vi "Periodic Tasks.vi"(8 "error constant":errorcluster) -> ()   [LabVIEW 2014]
doc: "This VI runs in parallel to other tasks. It can contain as many user-defined periodic loops as you need. These can carry out PID or other sorts of timed response."
uses:
  <vilib>/Rock Robotics/WPI/Solenoid/WPI_SolenoidValue.ctl
  Dashboard Project/DashboardToRobotCluster.ctl
  Robot Global Data.vi
  <vilib>/Rock Robotics/WPI/Solenoid/WPI_SolenoidSetEnum.vi
  <vilib>/Rock Robotics/WPI/RobotDrive/WPI_RobotDriveGetSetRefNum.vi
  <vilib>/Rock Robotics/WPI/RobotDrive/WPI_RobotDriveMecanumDrive_Cartesian.vi
  navX-MXP Library/navX-MXP IMU.lvlib
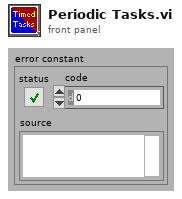
[diagram p1: front panel]
types:
  T1 = typedef "DashboardToRobotCluster.ctl" = cluster{"Test":dbl}
  T2 = typedef "WPI_SolenoidValue.ctl" = enum16{"Off", "On", "Forward", "Reverse"}
  T3 = cluster{"Front Right Motor":dbl, "Front Left Motor":dbl, "Rear Right Motor":dbl, "Rear Left Motor":dbl, "Current Heading":dbl, "Tote lift Up":bool, "Primary Feeder running":bool, "Secondary Feeder running":bool, "Totes In Robot":dbl, "Pressure In Tank":dbl, "Can Grabber State":T2}
  T4 = typedef "navX-MXP IMU.lvlib/navX SPI DevRef.ctl" = cluster{"SPIDevRef":T5, "Board Information":T8, "Status":T9, "Offsets":cluster{"Yaw":dbl, "Quat W":dbl, "Quat X":dbl, "Quat Y":dbl, "Quat Z":dbl}, "Update Rate (4Hz-60Hz)":u8, "refnum name":string, "error":errorcluster}
  T5 = typedef "WPI_SPIDevRef.ctl" = cluster{"DevStatus":errorcluster, "Handle":i32, "Controller":T6, "SPI Bus":T7}
  T6 = typedef "FPGA_TypedefDigitalModule.ctl" = enum16{"Controller 1"}
  T7 = typedef "spi_bus.ctl" = enum16{"SPI On-Board, CS0", "SPI On-Board, CS1", "SPI On-Board, CS2", "SPI On-Board, CS3", "SPI MXP", "Invalid"}
  T8 = typedef "navX-MXP IMU.lvlib/navX Board Information.ctl" = cluster{"WhoAmI (50 | 0x32)":u8, "Board Revision":u8, "Firmware Major Version":u8, "Firmware Minor Version":u8}
  T9 = typedef "navX-MXP IMU.lvlib/navX Status Data.ctl" = cluster{"Update Rate Hz":u8, "Accelerometer Full-Scale Range":u8, "Gyro Full-Scale Range":u16, "NAVX_OP_STATUS":T10, "NAVX_CAL_STATUS":T11, "NAVX_SELFTEST_STATUS":u8, "NAVX_SENSOR_STATUS":T12}
  T10 = typedef "navX-MXP IMU.lvlib/navX NAVX_OP_STATUS.ctl" = u8
  T11 = typedef "navX-MXP IMU.lvlib/navX NAVX_CAL_STATUS.ctl" = u8
  T12 = typedef "navX-MXP IMU.lvlib/navX NAVX_SENSOR_STATUS.ctl" = cluster{"MOVING":bool, "YAW_STABLE":bool, "MAG_DISTURBANCE":bool, "ALTITUDE_VALID":bool, "SEALEVEL_PRESS_SET":bool, "FUSED_HEADING_VALID":bool}
  T13 = typedef "WPI_RobotDriveDevRef.ctl" = cluster{"DevStatus":errorcluster, "Motors[]":T14[], "Square Inputs":bool, "Max Output":dbl}
  T14 = typedef "WPI_MotorControlDeviceRef.ctl" = cluster{"DeviceStatus":errorcluster, "Type":T15, "PWM":cluster{"Controller":T6, "PWM Channel":T16, "DeadBand":T17}, "CAN":cluster{"Device Number":u8, "Control Mode":T18, "Semaphore":T19, "Max Vout":dbl, "TalonSRX Control Mode":T20}, "Invert":bool, "TransformRef":T21, "InvTransformRef":T21}
  T15 = typedef "WPI_MotorControlType.ctl" = enum16{"PWM", "CAN", "CANTalonSRX"}
  T16 = typedef "FPGA_DIOPWMChannel.ctl" = enum8{"PWM 0", "PWM 1", "PWM 2", "PWM 3", "PWM 4", "PWM 5", "PWM 6", "PWM 7", "PWM 8", "PWM 9", "PWM MXP 0", "PWM MXP 1", "PWM MXP 2", "PWM MXP 3", "PWM MXP 4", "PWM MXP 5", "PWM MXP 6", "PWM MXP 7", "PWM MXP 8", "PWM MXP 9", "Invalid"}
  T17 = typedef "WPI_PWMDeadband.ctl" = cluster{"Name":string, "maxPositivePwm":i32, "minPositivePwm":i32, "centerPwm":i32, "maxNegativePwm":i32, "minNegativePwm":i32, "angularRange":u16}
  T18 = typedef "WPI_CANJaguar_ControlMode.ctl" = enum8{"Percent VBus", "Current", "Speed", "Position", "Voltage"}
  T19 = typedef "Semaphore RefNum" = refnum<k1>
  T20 = typedef "WPI_CANTalonSRX_APIControlMode.ctl" = enum8{"Percent VBus", "Speed", "Position", "Slave", "Unchanged / Invalid"}
  T21 = typedef "WPI_PWMTransform_ConPane.ctl" = refnum<vi>
  T22 = typedef "navX-MXP IMU.lvlib/navX YPRH Data.ctl" = cluster{"Yaw":dbl, "Pitch":dbl, "Roll":dbl, "Heading":dbl}
  T23 = typedef "WPI_SolenoidDevRef.ctl" = cluster{"DevStatus":errorcluster, "Pneumatics Control Module":u8, "Forward Solenoid Channel":T24, "Reverse Solenoid Channel":T24}
  T24 = typedef "WPI_SolenoidChannel.ctl" = enum8{"Solenoid 0", "Solenoid 1", "Solenoid 2", "Solenoid 3", "Solenoid 4", "Solenoid 5", "Solenoid 6", "Solenoid 7", "Invalid"}
  T25 = cluster{"Primary Infeed":dbl, "Secondary Infeed":dbl, "Lifter":bool}
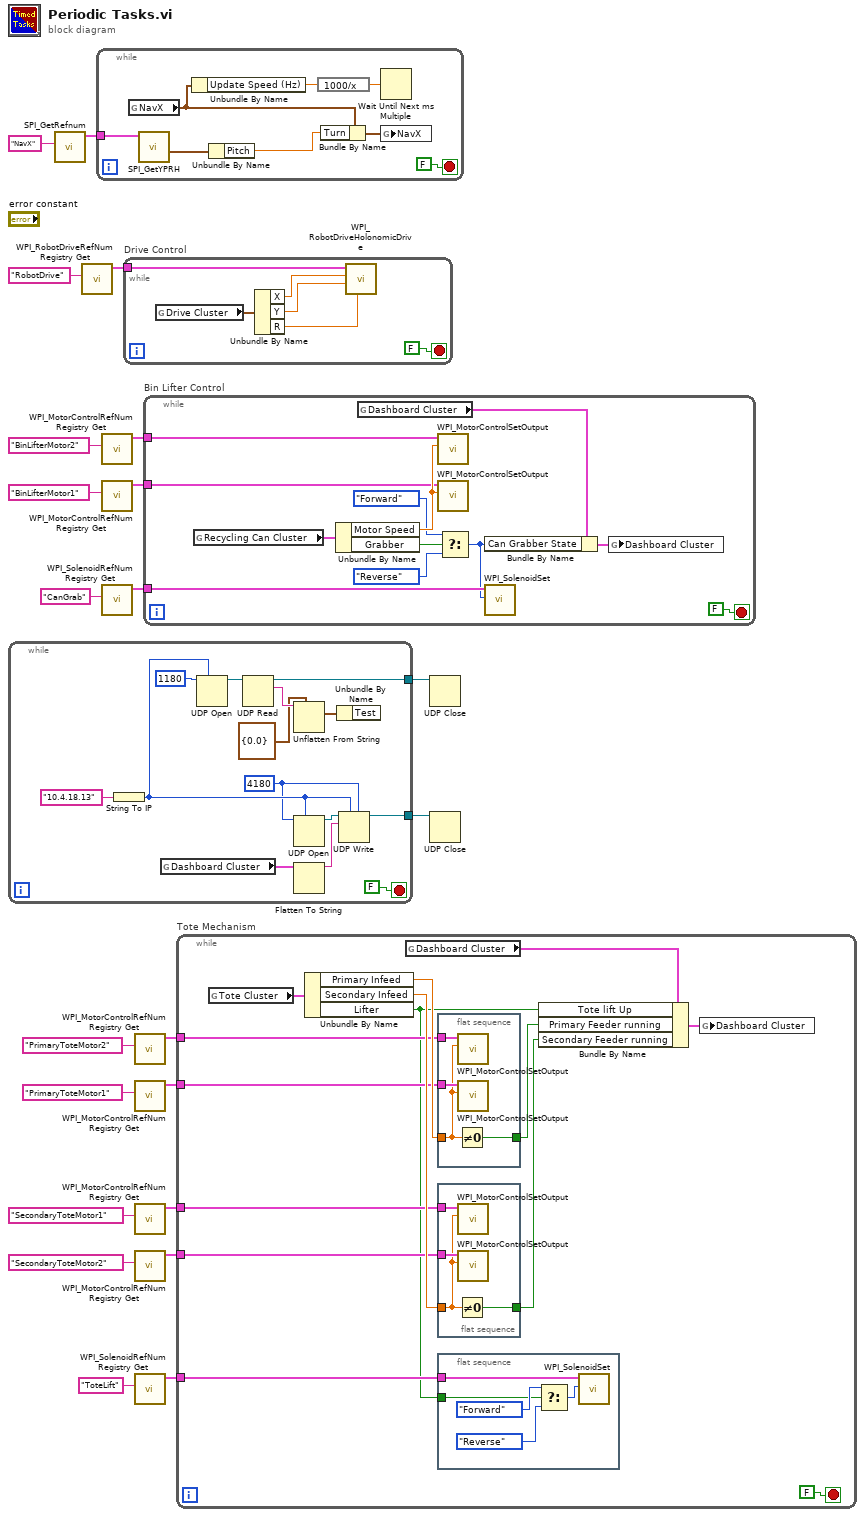
[diagram p0: block diagram]
diagram:
  n1 = while {
    tunnel: [w35] -> w22
    tunnel: [w34] -> w21
    stop <- FALSE stop-if-true
    w23 = u16 4180 ("port")
    n2 = String To IP(1:"10.4.18.13" ("name")) -> (0:w24:u32)
    n3 = global read "Robot Global Data.vi" "Dashboard Cluster"() -> (w32:T3)
    n4 = UDP Open(7:w24, 11:u16 1180 ("port")) -> (port=w26:refnum<k16>)  [unwired: 3 in, 2 out]
    n5 = UDP Read(connection ID=w26) -> (data out=w30:string, 3:w34:refnum<k16>)  [unwired: 3 in, 3 out]
    n6 = Unflatten From String(type=T1 {"Test"=0.0} ("Cluster"), binary string=w30) -> (value=w28:T1)  [unwired: 3 in, 2 out]
    n7 = UDP Open(7:w24, 11:w23) -> (port=w27:refnum<k16>)  [unwired: 3 in, 2 out]
    n8 = Flatten To String(anything=w32) -> (data string=w31:string)  [unwired: 3 in, 2 out]
    n9 = Unbundle By Name(w28) -> ()  [unwired: 1 out]
    n10 = UDP Write(address=w24, port or service name=w23, connection ID=w27, data in=w31) -> (3:w35:refnum<k16>)  [unwired: 2 in, 1 out]
  }
  n11 = call "SPI_GetRefnum.vi"("refnum name"="NavX") -> ("navX DevRef"=w1:T4)  [unwired: 9 in, 1 out]
  n12 = call <vilib>:"WPI_RobotDriveRefNum Registry Get.vi"("refnum name"="RobotDrive") -> ("RobotDriveDevRef"=w3:T13)  [unwired: 9 in, 1 out]
  n13 = while {
    tunnel: w1 -> [w43]
    stop <- FALSE stop-if-true
    n14 = global read "Robot Global Data.vi" "NavX"() -> (w41:cluster{"Update Speed (Hz)":dbl, "Turn":dbl})
    n15 = call "SPI_GetYPRH.vi"("navX DevRef"=w43) -> ("YPRH"=w38:T22)  [unwired: 8 in, 2 out]
    n16 = Unbundle By Name(w41) -> ("Update Speed (Hz)"=w40:dbl)
    n17 = Unbundle By Name(w38) -> ("Pitch"=w37:dbl)
    n18 = expression code="1000/x"(w40) -> (w39:dbl)
    n19 = Bundle By Name(cluster=w41, "Turn"=w37) -> (w42:cluster{"Update Speed (Hz)":dbl, "Turn":dbl})
    n20 = Wait Until Next ms Multiple(millisecond multiple=w39) -> ()  [unwired: 1 out]
    n21 = global write "Robot Global Data.vi" "NavX"(w42) -> ()
  }
  n22 = call <vilib>:"WPI_MotorControlRefNum Registry Get.vi"("refnum name"="BinLifterMotor2") -> ("MotorControlDevRef"=w9:T14)  [unwired: 9 in, 1 out]
  n23 = call <vilib>:"WPI_MotorControlRefNum Registry Get.vi"("refnum name"="BinLifterMotor1") -> ("MotorControlDevRef"=w7:T14)  [unwired: 9 in, 1 out]
  n24 = call <vilib>:"WPI_SolenoidRefNum Registry Get.vi"("refnum name"="CanGrab") -> ("SolenoidDevRef"=w5:T23)  [unwired: 9 in, 1 out]
  n25 = while "Drive Control" {
    tunnel: w3 -> [w45]
    stop <- FALSE stop-if-true
    n26 = global read "Robot Global Data.vi" "Drive Cluster"() -> (w49:cluster{"X":dbl, "Y":dbl, "R":dbl})
    n27 = Unbundle By Name(w49) -> ("X"=w48:dbl, "Y"=w47:dbl, "R"=w46:dbl)
    n28 = call-poly <vilib>:"WPI_RobotDriveHolonomicDrive.vi"("Rotation"=w46, "Y"=w47, "X"=w48, "RobotDriveDevRef"=w45) -> ()  [unwired: 5 in, 3 out]
  }
  n29 = call <vilib>:"WPI_MotorControlRefNum Registry Get.vi"("refnum name"="PrimaryToteMotor2") -> ("MotorControlDevRef"=w16:T14)  [unwired: 9 in, 1 out]
  n30 = call <vilib>:"WPI_MotorControlRefNum Registry Get.vi"("refnum name"="PrimaryToteMotor1") -> ("MotorControlDevRef"=w15:T14)  [unwired: 9 in, 1 out]
  n31 = call <vilib>:"WPI_MotorControlRefNum Registry Get.vi"("refnum name"="SecondaryToteMotor1") -> ("MotorControlDevRef"=w12:T14)  [unwired: 9 in, 1 out]
  n32 = call <vilib>:"WPI_MotorControlRefNum Registry Get.vi"("refnum name"="SecondaryToteMotor2") -> ("MotorControlDevRef"=w11:T14)  [unwired: 9 in, 1 out]
  n33 = call <vilib>:"WPI_SolenoidRefNum Registry Get.vi"("refnum name"="ToteLift") -> ("SolenoidDevRef"=w19:T23)  [unwired: 9 in, 1 out]
  n34 = while "Bin Lifter Control" {
    tunnel: w9 -> [w54]
    tunnel: w7 -> [w53]
    tunnel: w5 -> [w52]
    stop <- FALSE stop-if-true
    n35 = global read "Robot Global Data.vi" "Recycling Can Cluster"() -> (w60:cluster{"Motor Speed":dbl, "Grabber":bool})
    n36 = Unbundle By Name(w60) -> ("Motor Speed"=w61:dbl, "Grabber"=w57:bool)
    n37 = global read "Robot Global Data.vi" "Dashboard Cluster"() -> (w55:T3)
    n38 = call <vilib>:"WPI_MotorControlSetOutput.vi"("Output"=w61, "MotorControlDevRef"=w54) -> ()  [unwired: 7 in, 3 out]
    n39 = call <vilib>:"WPI_MotorControlSetOutput.vi"("Output"=w61, "MotorControlDevRef"=w53) -> ()  [unwired: 7 in, 3 out]
    n40 = Select(t=WPI_SolenoidValue."Forward" ("Value"), s=w57, f=WPI_SolenoidValue."Reverse" ("Value")) -> (s? t:f=w51:T2)
    n41 = Bundle By Name(cluster=w55, "Can Grabber State"=w51) -> (w56:T3)
    n42 = call-poly <vilib>:"WPI_SolenoidSet.vi"("Value"=w51, "SolenoidDevRef"=w52) -> ()  [unwired: 8 in, 2 out]
    n43 = global write "Robot Global Data.vi" "Dashboard Cluster"(w56) -> ()
  }
  n44 = while "Tote Mechanism" {
    tunnel: w19 -> [w70]
    tunnel: w16 -> [w69]
    tunnel: w15 -> [w68]
    tunnel: w12 -> [w67]
    tunnel: w11 -> [w66]
    stop <- FALSE stop-if-true
    n45 = global read "Robot Global Data.vi" "Tote Cluster"() -> (w73:T25)
    n46 = Unbundle By Name(w73) -> ("Primary Infeed"=w75:dbl, "Secondary Infeed"=w74:dbl, "Lifter"=w63:bool)
    n47 = global read "Robot Global Data.vi" "Dashboard Cluster"() -> (w71:T3)
    n48 = flat-sequence {
      tunnel: w75 -> [w87]
      tunnel: w69 -> [w89]
      tunnel: w68 -> [w88]
      tunnel: [w86] -> w65
      frame #0 {
        n49 = Not Equal To 0?(x=w87) -> (x != 0?=w86:bool)
        n50 = call <vilib>:"WPI_MotorControlSetOutput.vi"("Output"=w87, "MotorControlDevRef"=w89) -> ()  [unwired: 7 in, 3 out]
        n51 = call <vilib>:"WPI_MotorControlSetOutput.vi"("Output"=w87, "MotorControlDevRef"=w88) -> ()  [unwired: 7 in, 3 out]
      }
    }
    n52 = flat-sequence {
      tunnel: w74 -> [w83]
      tunnel: w67 -> [w85]
      tunnel: w66 -> [w84]
      tunnel: [w82] -> w64
      frame #0 {
        n53 = Not Equal To 0?(x=w83) -> (x != 0?=w82:bool)
        n54 = call <vilib>:"WPI_MotorControlSetOutput.vi"("Output"=w83, "MotorControlDevRef"=w85) -> ()  [unwired: 7 in, 3 out]
        n55 = call <vilib>:"WPI_MotorControlSetOutput.vi"("Output"=w83, "MotorControlDevRef"=w84) -> ()  [unwired: 7 in, 3 out]
      }
    }
    n56 = flat-sequence {
      tunnel: w70 -> [w81]
      tunnel: w63 -> [w77]
      frame #0 {
        n57 = Select(t=WPI_SolenoidValue."Forward" ("Value"), s=w77, f=WPI_SolenoidValue."Reverse" ("Value")) -> (s? t:f=w78:T2)
        n58 = call-poly <vilib>:"WPI_SolenoidSet.vi"("Value"=w78, "SolenoidDevRef"=w81) -> ()  [unwired: 8 in, 2 out]
      }
    }
    n59 = Bundle By Name(cluster=w71, "Tote lift Up"=w63, "Primary Feeder running"=w65, "Secondary Feeder running"=w64) -> (w72:T3)
    n60 = global write "Robot Global Data.vi" "Dashboard Cluster"(w72) -> ()
  }
  n61 = UDP Close(connection ID=w21) -> ()  [unwired: 1 in, 2 out]
  n62 = UDP Close(connection ID=w22) -> ()  [unwired: 1 in, 2 out]
